vi "sCMOS_init_ramp_FPGA.vi"(3 "error in":errorcluster, 4 "data cluster":T1, 5 "handle":u32) -> (0 "error out":errorcluster {"code" format="%.0x"}, 1 "Ready?":bool, 2 "Frames":i32)   [LabVIEW 2015]
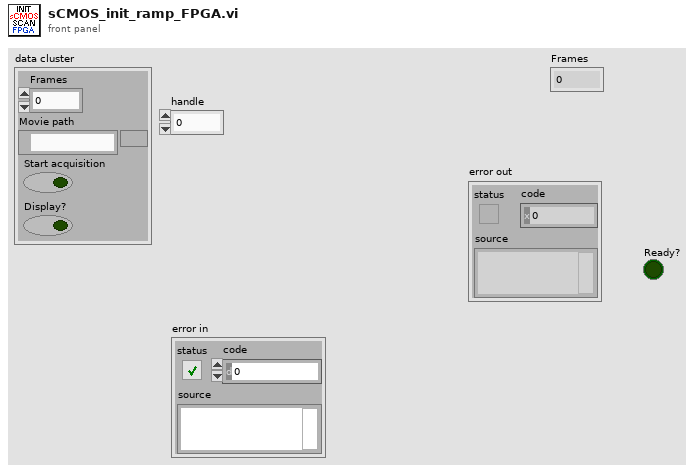
[diagram p1: front panel]
types:
  T1 = cluster{"Frames":i32, "Movie path":path, "Start acquisition":bool, "Display?":bool}
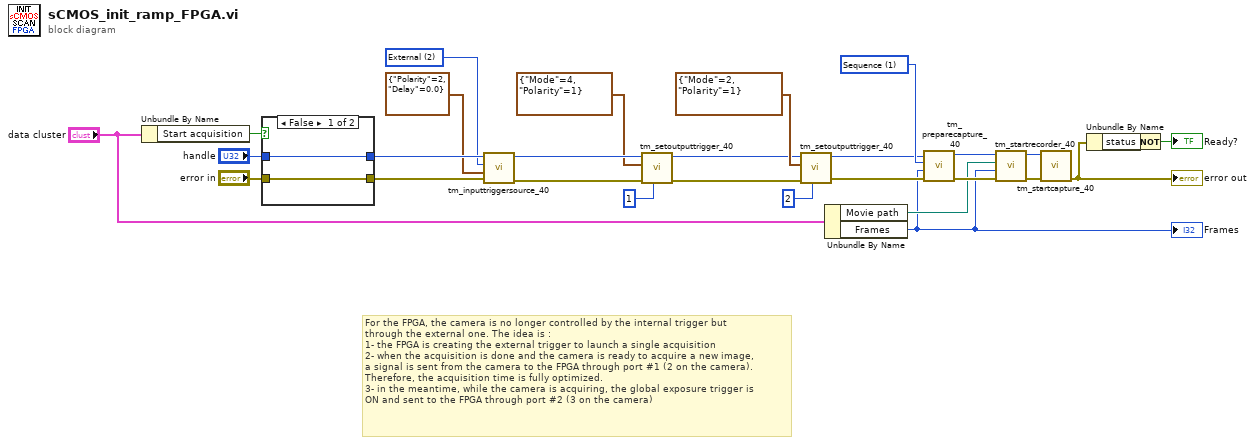
[diagram p0: block diagram]
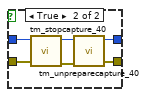
[diagram p2: hidden frame]
diagram:
  w14 = 2 items=["Internal"=1, "External"=2, "Software"=3, "Master Pulse"=4] ("Source")
  w24 = 1 items=["Snap", "Sequence"] ("Capture mode")
  # "For the FPGA, the camera is no longer controlled by the internal trigger but\nthrough the external one. The idea is :\n1- the FPGA is creating the external trigger to launch a single acquisition\n2- when the acquisition is done and the camera is ready to acquire a new image, \na signal is sent from the camera to the FPGA through port #1 (2 on the camera).\nTherefore, the acquisition time is fully optimized.\n3- in the meantime, while the camera is acquiring, the global exposure trigger is\nON and sent to the FPGA through port #2 (3 on the camera)"
  n1 = Unbundle By Name("data cluster") -> ("Start acquisition"=w21:bool)
  n2 = case shown="False" w21 {
    tunnel: "error in" -> [w30 w36]
    tunnel: [w30 w32] -> w15
    tunnel: "handle" -> [w29 w35]
    tunnel: [w29 w31] -> w16
    frame False {
    }
    frame True {
      n3 = call <userlib>:"tm_stopcapture_40.vi"("error in (no error)"=w36, "Handle in"=w35) -> ("error out"=w34:errorcluster, "Handle out"=w33:u32)  [unwired: 8 in]
      n4 = call <userlib>:"tm_unpreparecapture_40.vi"("error in (no error)"=w34, "Handle in"=w33) -> ("error out"=w32:errorcluster, "Handle out"=w31:u32)  [unwired: 8 in]
    }
  }
  n5 = call <userlib>:"tm_inputtriggersource_40.vi"("error in (no error)"=w15, "External Options"=cluster{"Polarity":i32, "Delay":dbl} {"Polarity"=2, "Delay"=0.0}, "Source"=w14, "Handle in"=w16) -> ("error out"=w11:errorcluster, "Handle out"=w12:u32)  [unwired: 6 in]
  n6 = call <userlib>:"tm_setoutputtrigger_40.vi"("Port"=1, "error in (no error)"=w11, "Type"=cluster{"Mode":u32, "Polarity":u32} {"Mode"=4, "Polarity"=1}, "Handle in"=w12) -> ("error out"=w5:errorcluster, "Handle out"=w6:u32)  [unwired: 6 in]
  n7 = call <userlib>:"tm_setoutputtrigger_40.vi"("Port"=2, "error in (no error)"=w5, "Type"=cluster{"Mode":u32, "Polarity":u32} {"Mode"=2, "Polarity"=1}, "Handle in"=w6) -> ("error out"=w3:errorcluster, "Handle out"=w4:u32)  [unwired: 6 in]
  n8 = Unbundle By Name("data cluster") -> ("Movie path"=w20:path, "Frames"=w2:i32)
  "Frames" <- w2
  n9 = call <userlib>:"tm_preparecapture_40.vi"("error in (no error)"=w3, "Frames"=w2, "Capture mode"=w24, "Handle in"=w4) -> ("error out"=w25:errorcluster, "Handle out"=w26:u32)  [unwired: 4 in, 2 out]
  n10 = call <userlib>:"tm_startrecorder_40.vi"("error in (no error)"=w25, "frames"=w2, "File"=w20, "Handle in"=w26) -> ("error out"=w27:errorcluster, "Handle out"=w28:u32)  [unwired: 6 in]
  n11 = call <userlib>:"tm_startcapture_40.vi"("error in (no error)"=w27, "Handle in"=w28) -> ("error out"=w19:errorcluster)  [unwired: 8 in, 1 out]
  "error out" <- w19
  n12 = Unbundle By Name(w19) -> ("status"=w18:bool)
  n13 = Not(x=w18) -> (.not. x?=→"Ready?":bool)
